vi "state.vi"() -> ()   [LabVIEW 2024]
uses:
  OneDrive - Embry-Riddle Aeronautical University/Admin/Facilities/TC3/TC3 DAC/Code/RTC_PXIe-Code v1_9_0 CODE/QMH-Architecture/support/Control/streamIO_states.ctl
panel:
  in  "Enum":T1=enum."Initialize"
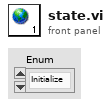
[diagram p1: front panel]
types:
  T1 = typedef "streamIO_states.ctl" = enum16{"Fault", "Initialize", "Stream", "Close"}
diagram:
